vi "Get Axis JSON Settings.vi"(0 "Graph In":refnum<class "Graph.lvclass">, 1 "Minimums":dbl[](array[numeric]), 2 "Maximums":dbl[](array[numeric]), 3 "Series JSON In":string, 5 "XYGraph Refnum":refnum<vi>, 7 "Plot Y Scale Index":u32[](array[numeric]), 9 "Value Only":bool, 11 "error in (no error)":errorcluster) -> (4 "X Axis Settings":string, 6 "Y Axis Settings":string, 10 "Series JSON Out":string, 15 "error out":errorcluster)   [LabVIEW 2017, in "Front Panel Publisher.lvlib" / "Graph.lvclass"]
uses:
  Graph.lvclass
  <userlib>/_OpenG.lib/array/array.llb/Remove Duplicates from 1D Array (U32)__ogtk.vi
  <userlib>/_OpenG.lib/array/array.llb/Index 1D Array Elements (String)__ogtk.vi
  <userlib>/_OpenG.lib/array/array.llb/Delete Elements from 1D Array (String)__ogtk.vi
  <userlib>/_OpenG.lib/array/array.llb/Remove Duplicates from 1D Array (I16)__ogtk.vi
  <userlib>/_OpenG.lib/array/array.llb/Conditional Auto-Indexing Tunnel (DBL)__ogtk.vi
  Front Panel Publisher.lvlib
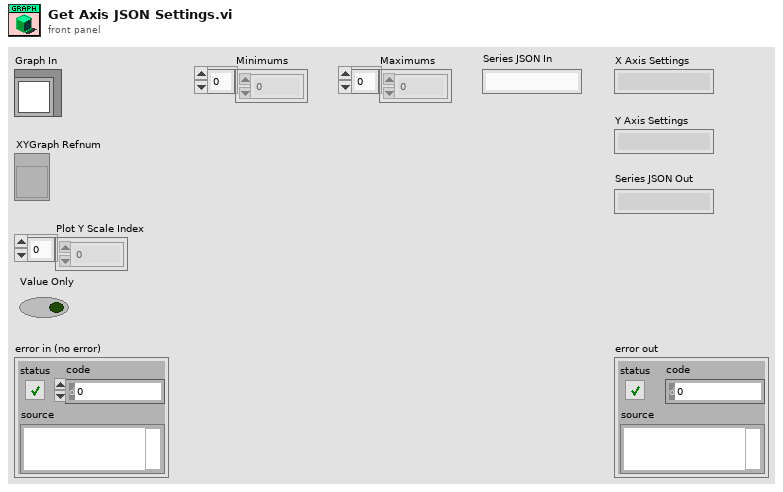
[diagram p1: front panel]
types:
  T1 = typedef "Front Panel Publisher.lvlib/Graph.lvclass/Attributes.ctl" = cluster{"X Label Text":string, "X Format String":string, "Y Label Text":string[], "Y Format String":string[], "Plot Y Axis Selection":enum16{"Y Axis", "Y2 Axis"}[], "Width":u32, "Series JSON Data":string}
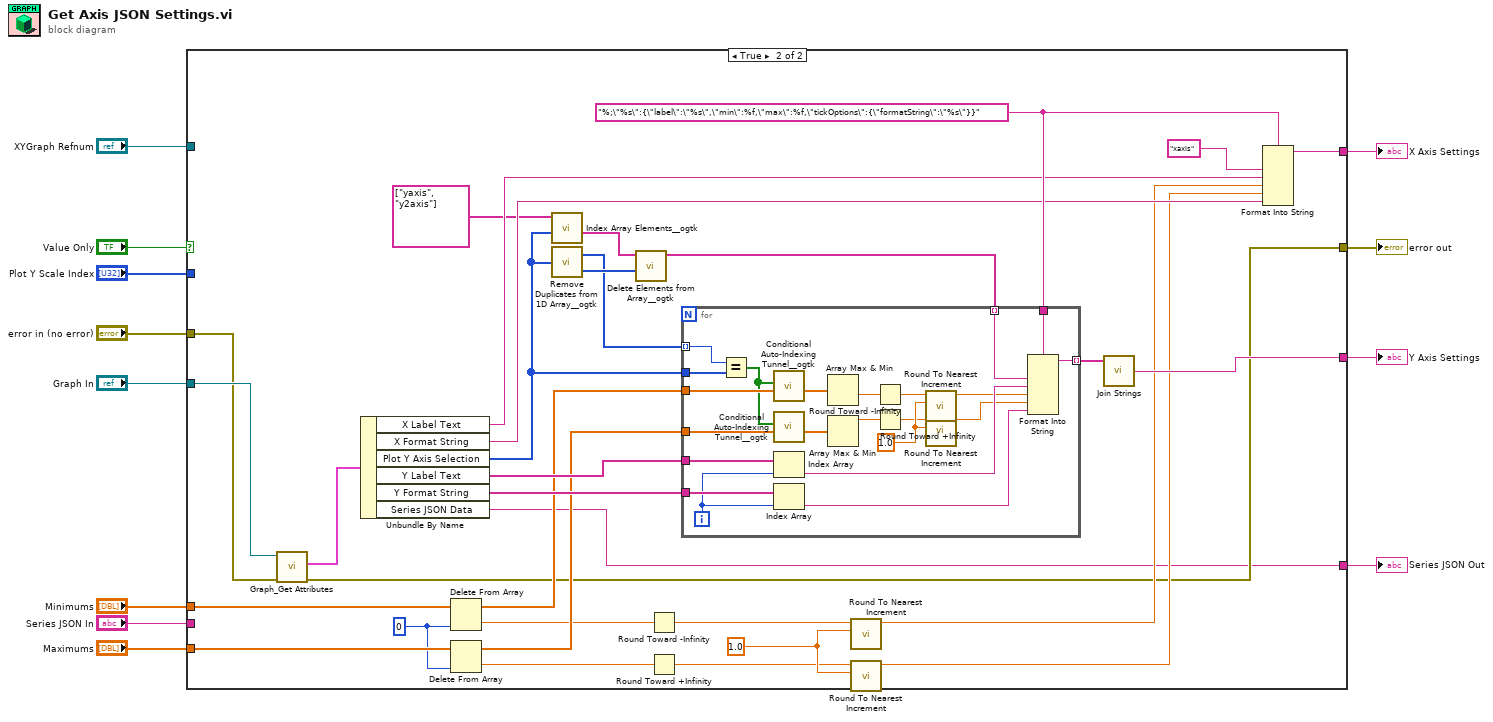
[diagram p0: block diagram]
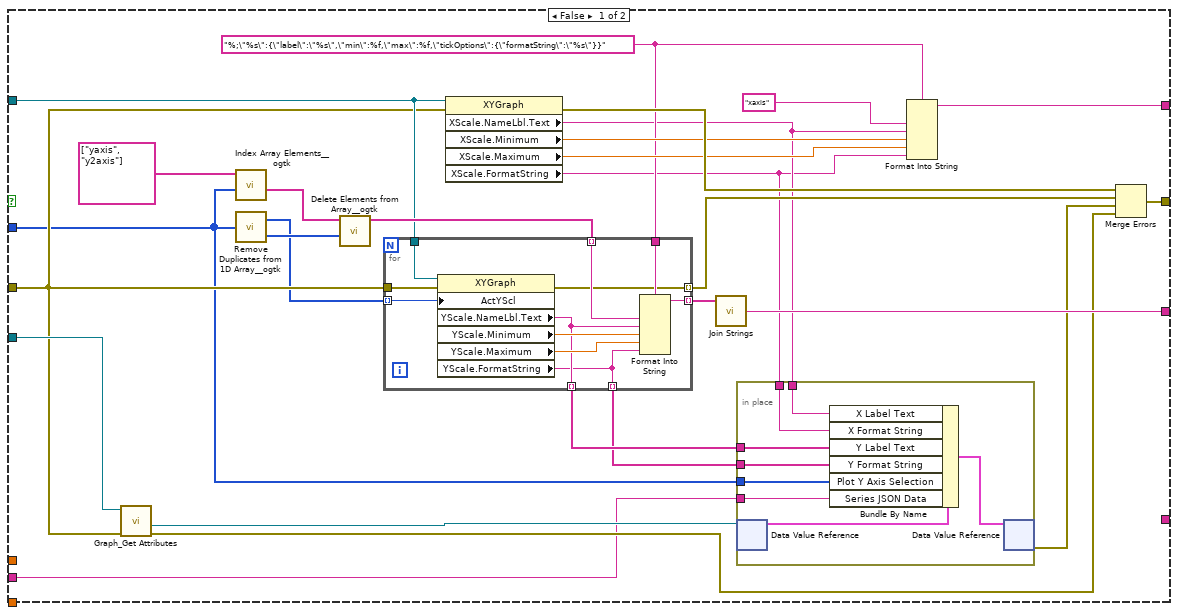
[diagram p2: hidden frame]
diagram:
  n1 = case shown="True" "Value Only" {
    tunnel: [w39 w63] -> w12
    tunnel: "Plot Y Scale Index" -> [w14 _]
    tunnel: [w33 w89] -> w10
    tunnel: [w30 w88] -> w9
    tunnel: "error in (no error)" -> [w20 w84]
    tunnel: "XYGraph Refnum" -> [w25 _]
    tunnel: "Graph In" -> [w24 w85]
    tunnel: "Maximums" -> [_ w78]
    tunnel: "Minimums" -> [_ w77]
    tunnel: [_ w59] -> w1
    tunnel: "Series JSON In" -> [w13 _]
    frame False {
      w26 = "%;\"%s\":{\"label\":\"%s\",\"min\":%f,\"max\":%f,\"tickOptions\":{\"formatString\":\"%s\"}}"
      n2 = call "Graph_Get Attributes.vi"("error in (no error)"=w20, "reference in"=w24) -> ("error out"=w18:errorcluster, "Graph DVR"=w23:refnum<data-value>)  [unwired: 6 in, 2 out]
      n3 = call-poly <userlib>:"Index Array Elements__ogtk.vi"("indices"=w14, "array"=string[] ["yaxis", "y2axis"]) -> ("elements"=w36:string[])  [unwired: 9 in]
      n4 = call-poly <userlib>:"Remove Duplicates from 1D Array__ogtk.vi"("Input Array"=w14) -> ("Output Array"=w15:u32[], "indices of removed elements"=w28:i32[])
      n5 = call-poly <userlib>:"Delete Elements from Array__ogtk.vi"("indices"=w28, "array"=w36) -> ("array w/ subset deleted"=w27:string[])  [unwired: 8 in, 1 out]
      n6 = for {
        tunnel: w15 -> [w57] mode=indexing
        tunnel: w27 -> [w56] mode=indexing
        tunnel: [w53] -> w34 mode=indexing
        tunnel: w26 -> [w52]
        tunnel: w25 -> [w51]
        tunnel: w20 -> [w58]
        tunnel: [w50] -> w38 mode=indexing
        tunnel: [w49] -> w17 mode=indexing
        tunnel: [w48] -> w16 mode=indexing
        n7 = property on="Property Node" class="XYGraph"(reference=w51, error in=w58, "ActYScl"=w57) -> (error out=w50:errorcluster, "YScale.NameLbl.Text"=w49:string, "YScale.Minimum"=w55:dbl, "YScale.Maximum"=w54:dbl, "YScale.FormatString"=w48:string)  [unwired: 1 out]
        n8 = Format Into String(format string=w52, w56, w49, w55, w54, w48) -> (resulting string=w53:string)  [unwired: 2 in, 1 out]
      }
      n9 = property on="Property Node" class="XYGraph"(reference=w25, error in=w20) -> (error out=w37:errorcluster, "XScale.NameLbl.Text"=w22:string, "XScale.Minimum"=w32:dbl, "XScale.Maximum"=w31:dbl, "XScale.FormatString"=w21:string)  [unwired: 1 out]
      n10 = call <vilib>:"Join Strings.vi"("Strings In"=w34) -> ("String"=w33:string)  [unwired: 2 in]
      n11 = in-place {
        in-place-border: w22 -> [w46]
        in-place-border: w21 -> [w45]
        in-place-border: w14 -> [w44]
        in-place-border: w17 -> [w42]
        in-place-border: w16 -> [w41]
        in-place-border: w13 -> [w40]
        n12 = in-place-dvr #1(w23) -> (w47:T1)  [unwired: 1 out]
        n13 = Bundle By Name(cluster=w47, "X Label Text"=w46, "X Format String"=w45, "Y Label Text"=w42, "Y Format String"=w41, "Plot Y Axis Selection"=w44, "Series JSON Data"=w40) -> (w43:T1)
        n14 = in-place-dvr #1(w43) -> (w19:errorcluster)  [unwired: 1 out]
      }
      n15 = Format Into String(format string=w26, "xaxis", w22, w32, w31, w21) -> (resulting string=w30:string)  [unwired: 2 in, 1 out]
      n16 = Merge Errors(w37, w38, w19, w18) -> (w39:errorcluster)
    }
    frame True {
      w62 = 0 ("index")
      w65 = 1.0 ("Increments to round")
      w86 = "%;\"%s\":{\"label\":\"%s\",\"min\":%f,\"max\":%f,\"tickOptions\":{\"formatString\":\"%s\"}}"
      n17 = call "Graph_Get Attributes.vi"("error in (no error)"=w84, "reference in"=w85) -> ("error out"=w63:errorcluster, "Graph Attributes"=w83:T1)  [unwired: 6 in, 2 out]
      n18 = Unbundle By Name(w83) -> ("X Label Text"=w82:string, "X Format String"=w81:string, "Plot Y Axis Selection"=w64:enum16{"Y Axis", "Y2 Axis"}[], "Y Label Text"=w80:string[], "Y Format String"=w79:string[], "Series JSON Data"=w59:string)
      n19 = Delete From Array(array=w77, index=w62) -> (deleted portion=w67:dbl, array with subset deleted=w71:dbl[])  [unwired: 1 in]
      n20 = Delete From Array(array=w78, index=w62) -> (deleted portion=w66:dbl, array with subset deleted=w70:dbl[])  [unwired: 1 in]
      n21 = call-poly <userlib>:"Index Array Elements__ogtk.vi"("indices"=w64, "array"=string[] ["yaxis", "y2axis"]) -> ("elements"=w76:string[])  [unwired: 9 in]
      n22 = call-poly <userlib>:"Remove Duplicates from 1D Array__ogtk.vi"("Input Array"=w64) -> ("Output Array"=w72:i16[], "indices of removed elements"=w75:i32[])
      n23 = call-poly <userlib>:"Delete Elements from Array__ogtk.vi"("indices"=w75, "array"=w76) -> ("array w/ subset deleted"=w73:string[])  [unwired: 8 in, 1 out]
      n24 = Round Toward -Infinity(1:w67) -> (0:w61:dbl)
      n25 = Round Toward +Infinity(x=w66) -> (ceil(x): smallest int >= x=w60:dbl)
      n26 = for {
        tunnel: w72 -> [w104] mode=indexing
        tunnel: w73 -> [w112] mode=indexing
        tunnel: [w111] -> w90 mode=indexing
        tunnel: w86 -> [w110]
        tunnel: w80 -> [w109]
        tunnel: w79 -> [w107]
        tunnel: w71 -> [w102]
        tunnel: w70 -> [w101]
        tunnel: w64 -> [w103]
        i -> [w105]
        w93 = 1.0 ("Increments to round")
        n27 = Equal?(x=w104, y=w103) -> (x = y?=w100:bool[])
        n28 = call-poly <userlib>:"Conditional Auto-Indexing Tunnel__ogtk.vi"("Array in"=w102, "Elements to keep"=w100) -> ("Filtered Array out"=w99:dbl[])  [unwired: 5 in]
        n29 = call-poly <userlib>:"Conditional Auto-Indexing Tunnel__ogtk.vi"("Array in"=w101, "Elements to keep"=w100) -> ("Filtered Array out"=w98:dbl[])  [unwired: 5 in]
        n30 = Index Array(array=w109, index=w105) -> (element=w108:string)
        n31 = Index Array(array=w107, index=w105) -> (element=w106:string)
        n32 = Array Max & Min(array=w99) -> (min value=w95:dbl)  [unwired: 3 out]
        n33 = Array Max & Min(array=w98) -> (max value=w94:dbl)  [unwired: 3 out]
        n34 = Round Toward -Infinity(1:w95) -> (0:w92:dbl)
        n35 = Round Toward +Infinity(x=w94) -> (ceil(x): smallest int >= x=w91:dbl)
        n36 = call "Round To Nearest Increment.vi"("Increments to round"=w93, "Number"=w92) -> ("Rounded Number"=w97:dbl)  [unwired: 9 in]
        n37 = call "Round To Nearest Increment.vi"("Increments to round"=w93, "Number"=w91) -> ("Rounded Number"=w96:dbl)  [unwired: 9 in]
        n38 = Format Into String(format string=w110, w112, w108, w97, w96, w106) -> (resulting string=w111:string)  [unwired: 2 in, 1 out]
      }
      n39 = call "Round To Nearest Increment.vi"("Increments to round"=w65, "Number"=w61) -> ("Rounded Number"=w69:dbl)  [unwired: 9 in]
      n40 = call "Round To Nearest Increment.vi"("Increments to round"=w65, "Number"=w60) -> ("Rounded Number"=w68:dbl)  [unwired: 9 in]
      n41 = call <vilib>:"Join Strings.vi"("Strings In"=w90) -> ("String"=w89:string)  [unwired: 2 in]
      n42 = Format Into String(format string=w86, "xaxis", w82, w69, w68, w81) -> (resulting string=w88:string)  [unwired: 2 in, 1 out]
    }
  }
  "error out" <- w12
  "Y Axis Settings" <- w10
  "X Axis Settings" <- w9
  "Series JSON Out" <- w1
